vi "ServotoPWMPulseWidth.vi"(8 "freq [Hz]":dbl, 10 "Pulse Width":dbl) -> (0 "Duty Cycle":dbl, 1 "Duty Cycle %":dbl, 2 "Pulse Width":dbl)   [LabVIEW 2013]
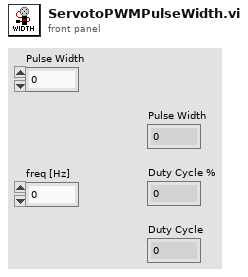
[diagram p1: front panel]
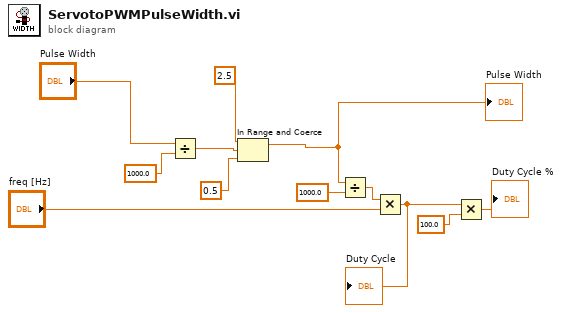
[diagram p0: block diagram]
diagram:
  n1 = Divide(x="Pulse Width", y=1000.0) -> (x/y=w5:dbl)
  n2 = In Range and Coerce(upper limit=2.5, x=w5, lower limit=0.5) -> (coerced(x)=w6:dbl)  [unwired: 1 out]
  "Pulse Width" <- w6
  n3 = Divide(x=w6, y=1000.0) -> (x/y=w9:dbl)
  n4 = Multiply(x=w9, y="freq [Hz]") -> (x*y=w12:dbl)
  "Duty Cycle" <- w12
  n5 = Multiply(x=w12, y=100.0) -> (x*y=→"Duty Cycle %":dbl)
